vi "fgt get differential Pressure.vi"(8 "error in (no error)":errorcluster, 11 "sensorIndex":u32) -> (0 "error out":errorcluster, 3 "value out":sgl)   [LabVIEW 2016, in "fgt_SDK.lvlib"]
doc: "Returns the current differential pressure measurement in mbar. This feature is only available on NIFS devices."
uses:
  fgt_SDK.lvlib
  dlls/fgt_SDK_32.dll
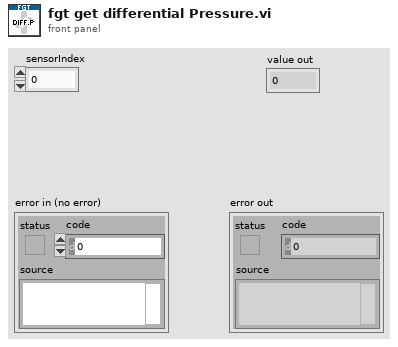
[diagram p1: front panel]
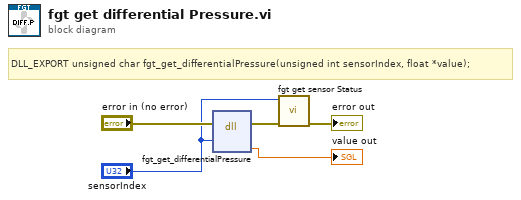
[diagram p0: block diagram]
diagram:
  # "DLL_EXPORT unsigned char fgt_get_differentialPressure(unsigned int sensorIndex, float *value);"
  n1 = dll-call lib="C:/projects/SDK/fgt-sdk-labview/dlls/fgt_SDK_*.*" fn="fgt_get_differentialPressure"(error in="error in (no error)", "sensorIndex"="sensorIndex") -> (error out=w3:errorcluster, "value"=→"value out":sgl)  [unwired: 5 in, 1 out]
  n2 = call "fgt get sensor Status.vi"("error in (no error)"=w3, "pressureIndex"="sensorIndex") -> ("error out"=→"error out":errorcluster)  [unwired: 9 in]
